vi "Scan_Stationary.vi"(8 "Error In":errorcluster, 9 "Scan Interval":dbl=1.0, 10 "Cluster Count":dbl=1.0, 11 "Number of Scans":dbl) -> (0 "Error Out":errorcluster, 3 "XY Graph":cluster{"X":dbl, "Y":dbl}[](graph))   [LabVIEW 2016, in "Hokuyo_URG.lvlib"]
uses:
  Hokuyo_URG.lvlib
  <instrlib>/Hokuyo URG Series/Public/Initialize-Standard.vi
  <instrlib>/Hokuyo URG Series/Hokuyo URG Series.lvlib
panel:
  in  "VISA resource name":refnum<visa-resource-name>="COM3"
  in  "stop":bool
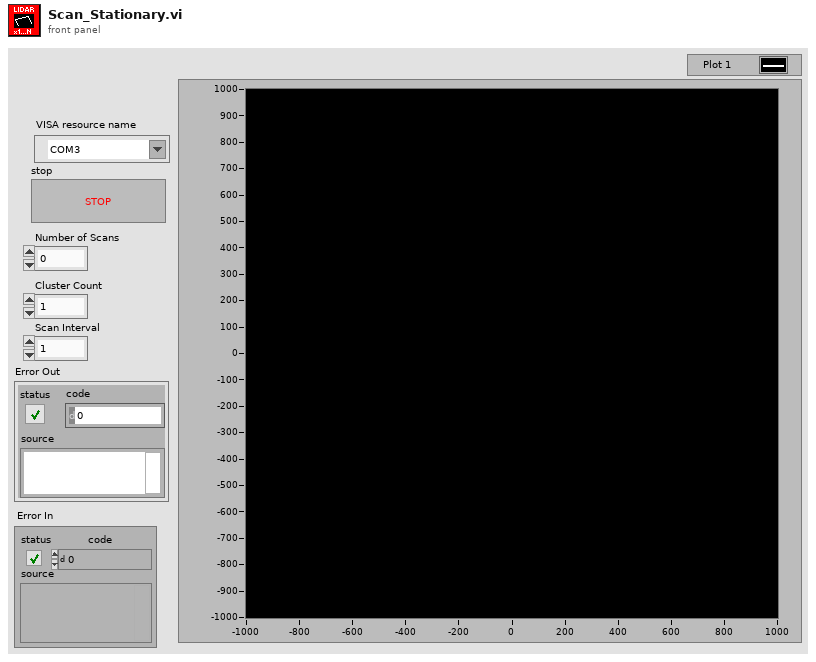
[diagram p1: front panel]
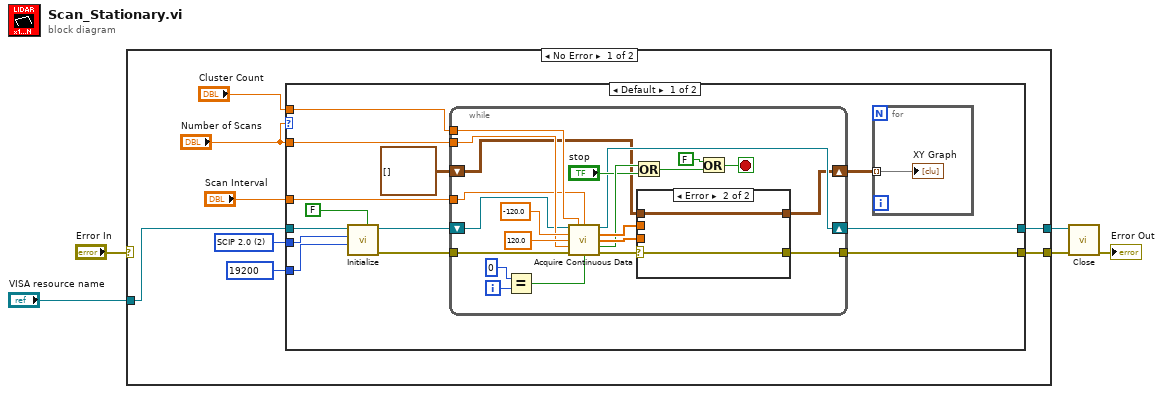
[diagram p0: block diagram]
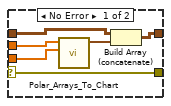
[diagram p2: hidden frame]
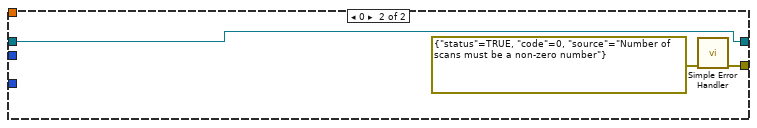
[diagram p3: hidden frame]
diagram:
  n1 = case shown="No Error" "Error In" {
    selector: "Error In" -> [_ w62]
    tunnel: [w11 w62] -> w5
    tunnel: "VISA resource name" -> [w7 w61]
    tunnel: [w6 w61] -> w2
    frame No Error {
      w12 = u32 19200 items=["19200"=19200, "57600"=57600, "115200"=115200, "250000"=250000, "500000"=500000, "750000"=750000] ("Serial Configuration (19200 : 19200 Baud)")
      w13 = u32 2 items=["Convert to Latest", "SCIP 1.1", "SCIP 2.0"] ("Protocol (2: SCIP 2.0)")
      n2 = case shown="Default" "Number of Scans" {
        tunnel: w7 -> [w26 w58]
        tunnel: w13 -> [w25 _]
        tunnel: w12 -> [w24 _]
        tunnel: [w22 w59] -> w11
        tunnel: "Number of Scans" -> [w21 _]
        tunnel: "Cluster Count" -> [w20 _]
        tunnel: "Scan Interval" -> [w19 _]
        tunnel: [w16 w58] -> w6
        frame Default {
          n3 = call-poly <instrlib>:"Initialize.vi"("Reset? (F: No)"=FALSE, "Serial Configuration (19200 : 19200 Baud)"=w24, "Protocol (2: SCIP 2.0)"=w25, "VISA resource name"=w26) -> ("error out"=w23:errorcluster, "VISA resource name out"=w18:refnum<visa-resource-name>)  [unwired: 6 in]
          n4 = while {
            tunnel: w23 -> [w48]
            tunnel: [w49] -> w22
            tunnel: w21 -> [w45]
            tunnel: w20 -> [w44]
            tunnel: w19 -> [w43]
            shift-right: [w37] -> w16
            shift-left: w18 -> [w36]
            shift-right: [w28] -> w15
            shift-left: cluster{"x":dbl, "y":dbl}[][] [] -> [w32]
            i -> [w34]
            stop <- w30 stop-if-true
            n5 = Equal?(x=0, y=w34) -> (x = y?=w33:bool)
            n6 = call <instrlib>:"Acquire Continuous Data.vi"("VISA resource name"=w36, "Cluster Count (1)"=w44, "Scan Interval (1)"=w43, "Start Point (-120°)"=-120.0, "End Point (120°)"=120.0, "Number of Scans (0)"=w45, "error in (no error)"=w48, "Enable Request Message (F:Disable)"=w33) -> ("VISA resource name out"=w37:refnum<visa-resource-name>, "Magnitude"=w41:dbl[], "Direction"=w40:dbl[], "Scan Ended?"=w39:bool, "error out"=w42:errorcluster)  [unwired: 2 in, 1 out]
            n7 = Or(x=w39, y="stop") -> (x .or. y?=w31:bool)
            n8 = case shown="Error" w42 {
              selector: w42 -> [w55 w57]
              tunnel: [w55 w57] -> w49
              tunnel: w41 -> [w54 _]
              tunnel: w40 -> [w53 _]
              tunnel: [w51 w56] -> w28
              tunnel: w32 -> [w52 w56]
              frame No Error {
                n9 = call "Polar_Arrays_To_Chart.vi"("Direction"=w53, "Magnitude"=w54) -> ("Scan"=w50:cluster{"x":dbl, "y":dbl}[])  [unwired: 7 in, 2 out]
                n10 = Build Array (concatenate)(w52, w50) -> (w51:cluster{"x":dbl, "y":dbl}[][])
              }
              frame Error {
              }
            }
            n11 = Or(x=FALSE ("reset"), y=w31) -> (x .or. y?=w30:bool)
          }
          n12 = for {
            tunnel: w15 -> [w27] mode=indexing
            "XY Graph" <- w27
          }
        }
        frame 0 {
          n13 = call <vilib>:"Simple Error Handler.vi"("error in (no error)"=errorcluster {"status"=TRUE, "code"=0, "source"="Number of scans must be a non-zero number"} ("error IO")) -> ("error out"=w59:errorcluster)  [unwired: 4 in, 4 out]
        }
      }
    }
    frame Error {
    }
  }
  n14 = call <instrlib>:"Close.vi"("error in (no error)"=w5, "VISA resource name"=w2) -> ("error out"=→"Error Out":errorcluster)  [unwired: 9 in]
